vi "RRAM.vi"(5 "Other Fixed Voltage (V)":dbl=2.0, 7 "Pulse Width (us)":dbl=100.0, 8 "Mode":T1(tab), 9 "Stride":u16=1, 10 "Final address":u16, 11 "Initial address":u16) -> ()   [LabVIEW 2019]
uses:
  <vilib>/Utility/file.llb/Read Delimited Spreadsheet (I64).vi
  Globals.vi
  <vilib>/Utility/file.llb/Write Delimited Spreadsheet (DBL).vi
panel:
  in  "Addr hold time (s)":dbl=0.0005 caption="Time Target (s)" format="%#_6p"
  out "Current address":i32
  in  "FORM outfile":path=path "C:/Users/Murmann-Group/Documents/LabVIEW Data/NI-RRAM-Test-Setup/form.csv"
  out "FORM resistance (ohm)":dbl format="%#_6p"
  out "FORM WL voltage (V)":dbl
  out "FORM BL voltage (V)":dbl
  out "formed?":bool
  in  "SET target resistance (ohm)":dbl format="%#_6p"
  out "SET resistance (ohm)":dbl format="%#_6p"
  out "SET WL voltage (V)":dbl
  out "SET BL voltage (V)":dbl
  out "set?":bool
  in  "SET outfile":path=path "C:/Users/Murmann-Group/Documents/LabVIEW Data/NI-RRAM-Test-Setup/set.csv"
  in  "RESET target resistance (ohm)":dbl=50000.0 format="%#_6p"
  in  "RESET outfile":path=path "C:/Users/Murmann-Group/Documents/LabVIEW Data/NI-RRAM-Test-Setup/reset.csv"
  out "reset?":bool
  out "RESET SL voltage (V)":dbl
  out "RESET WL voltage (V)":dbl
  out "RESET resistance (ohm)":dbl format="%#_6p"
  in  "number of samples":i32=500
  in  "voltage level (V)":dbl=0.2 format="%#_6p"
  in  "settling time (s)":dbl=0.002 caption="Time Target (s)" format="%#_6p"
  in  "READ outfile":path=path "C:/Users/Murmann-Group/Documents/LabVIEW Data/NI-RRAM-Test-Setup/read.csv"
  out "read voltages (V)":dbl[](array[numeric]) format="%#_6p"
  out "currents (A)":dbl[](array[numeric]) format="%#_6p"
  out "resistances (ohm)":dbl[](array[numeric]) format="%#_6p"
  in  "Sweep Type":T2(ring)
  in  "Sweep outfile":path=path "C:/Users/Murmann-Group/Documents/LabVIEW Data/NI-RRAM-Test-Setup/sweep-vwl-set.csv"
  in  "Target infile":path=path "C:/Users/RSG/Desktop/NI-Skywater-Test-Setup/target.csv"
  in  "Target from file?":bool
  in  "Upper resistance (ohm)":dbl=50000.0 format="%#_6p"
  in  "Lower resistance (ohm)":dbl=40000.0 format="%#_6p"
  in  "Retention outfile":path=path "C:/Users/RSG/Desktop/NI-Skywater-Test-Setup/target.csv"
  in  "Perform retention test":bool
  out "target final resistance (ohm)":dbl format="%#_6p"
  out "target hit?":bool
  out "Current target (from file)":i64
  in  "Target outfile":path=path "C:/Users/RSG/Desktop/NI-Skywater-Test-Setup/target.csv"
  in  "CB type":u16(ring)=1 items=["1 bit/cell"=1, "2 bit/cell"=2, "3 bit/cell"=3, "4 bit/cell"=4]
  in  "Read Ranges (multi-bit)":dbl[](array[numeric])=[0.0, 7000.0, 28000.0, 85000.0, 1000000000.0] format="%#_6p"
  in  "Write Targets (multi-bit)":dbl[][](array[numeric])=[[0.0, 6000.0], [20000.0, 25000.0], [70000.0, 75000.0], [140000.0, 500000.0]] format="%#_6p"
  in  "Read Ranges (1b)":dbl[](array[numeric])=[0.0, 7000.0, 1000000000.0] format="%#_6p"
  in  "Write Targets (1b)":dbl[][](array[numeric])=[[9000.0, 11000.0], [100000.0, 10000000000.0]] format="%#_6p"
  in  "CB size":i32=32
  in  "CB offset":i32
  out "Checkerboard":T3(plugin-control)
  out "Confusion Matrix":i32[][](array[numeric])
  out "BER":dbl
  in  "endurance file":path
  in  "Cycles":i32
  # "Checkerboard Write"
  # "Checkerboard Read"
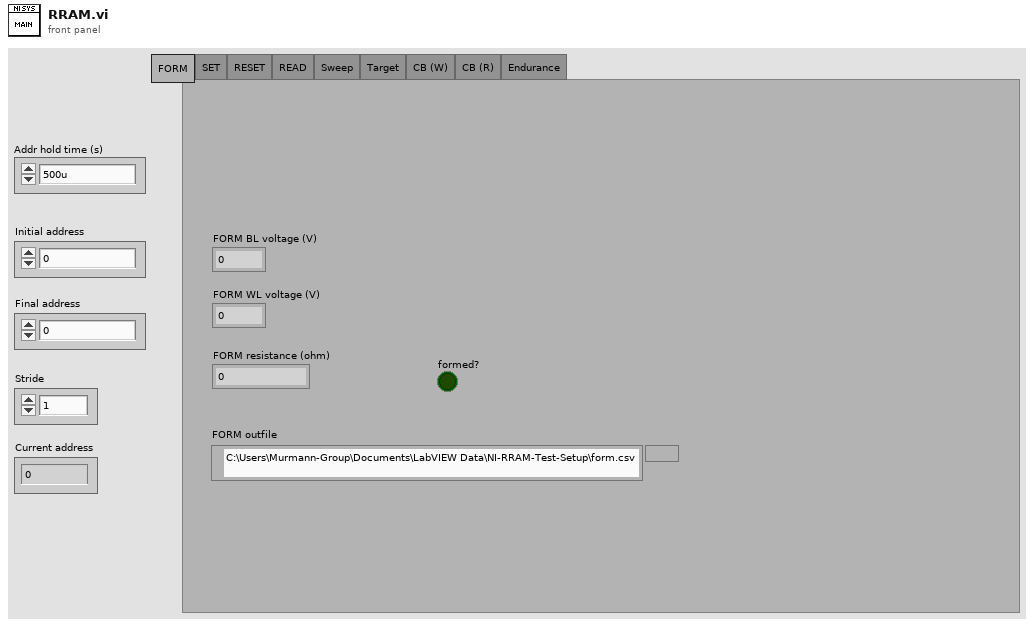
[diagram p1: front panel]
types:
  T1 = enum32{"FORM", "SET", "RESET", "READ", "Sweep", "Target", "CB (W)", "CB (R)", "Endurance"}
  T2 = enum16{"Sweep VWL SET", "Sweep VBL SET", "Sweep VWL RESET", "Sweep VSL RESET"}
  T3 = typedef "IMAQ Image.ctl" = refnum<image>
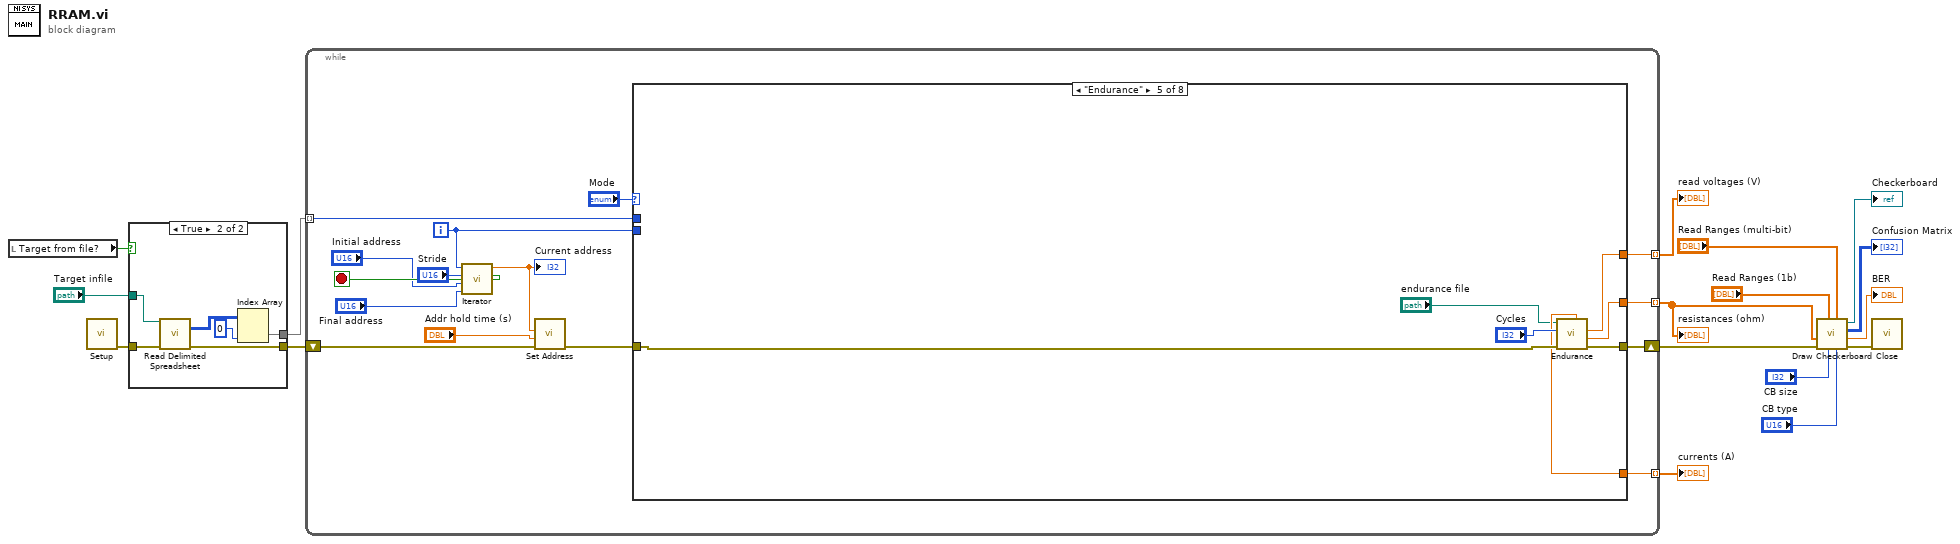
[diagram p0: block diagram]
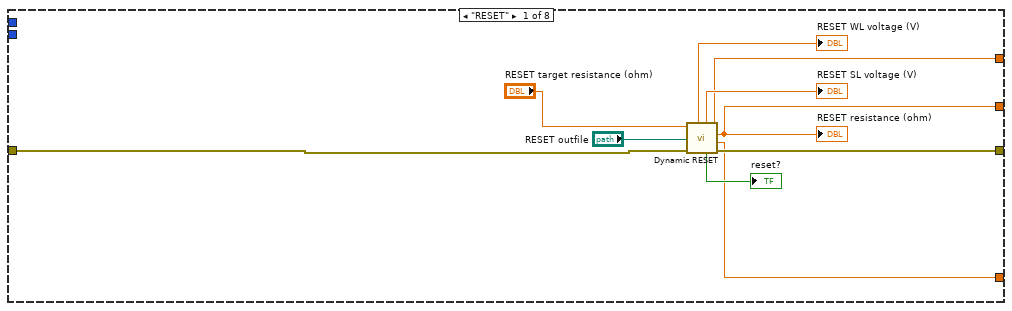
[diagram p3: hidden frame]
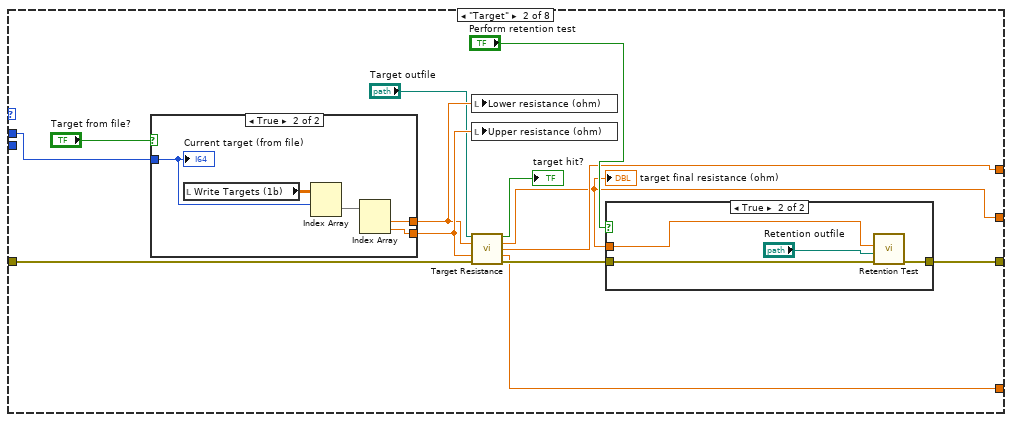
[diagram p4: hidden frame]
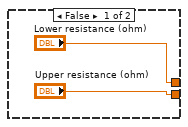
[diagram p5: hidden frame]
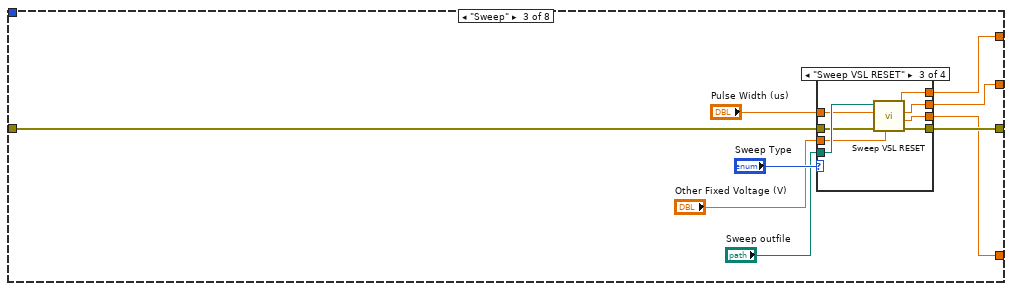
[diagram p7: hidden frame]
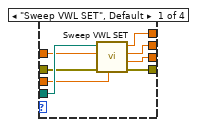
[diagram p8: hidden frame]
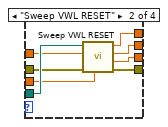
[diagram p9: hidden frame]
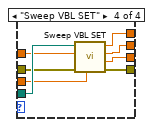
[diagram p10: hidden frame]
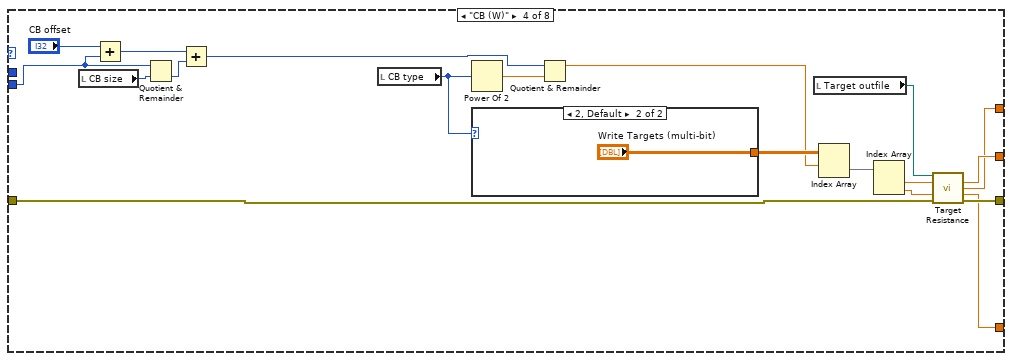
[diagram p11: hidden frame]
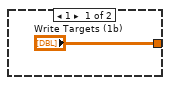
[diagram p12: hidden frame]
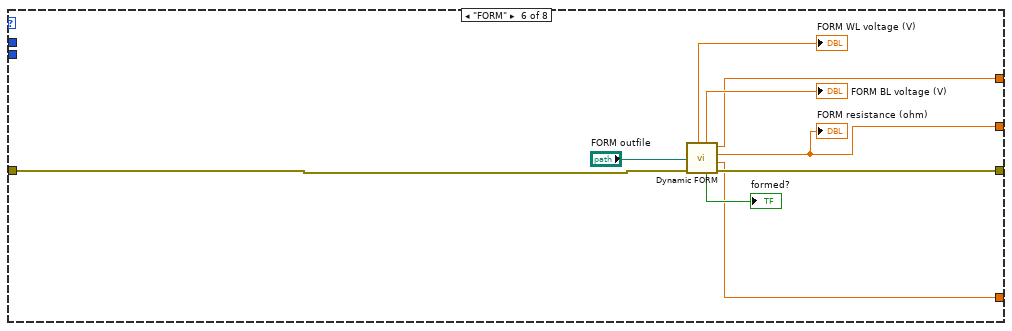
[diagram p13: hidden frame]
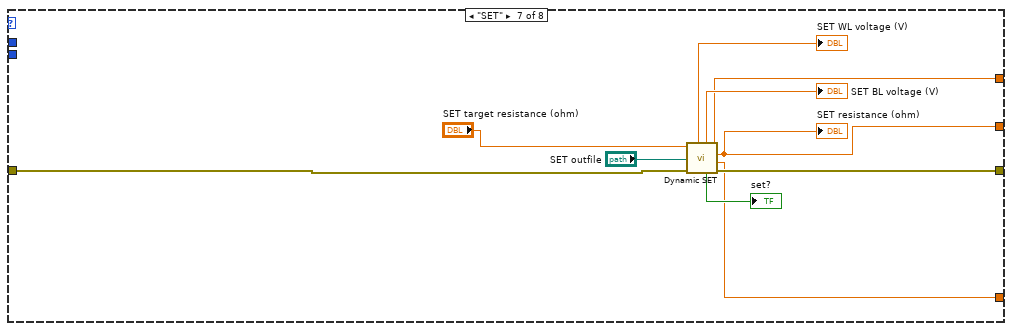
[diagram p14: hidden frame]
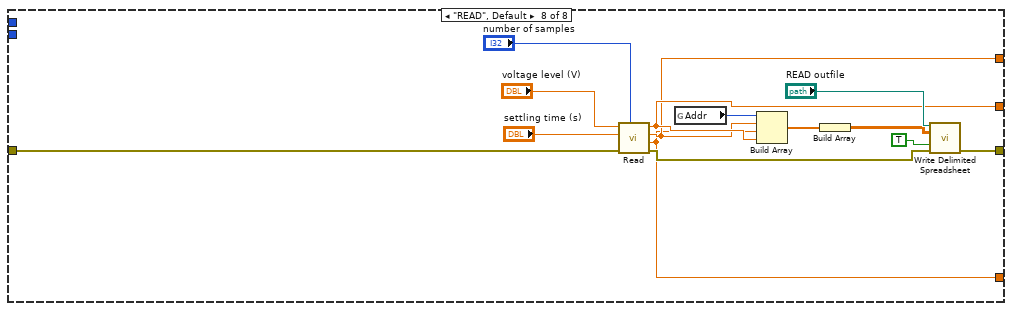
[diagram p15: hidden frame]
diagram:
  n1 = local read "Target from file?"() -> (w1:bool)
  n2 = call "Setup.vi"() -> ("error out"=w5:errorcluster)  [unwired: 10 in]
  n3 = case shown="True" w1 {
    tunnel: w5 -> [w18 w24]
    tunnel: [w18 w23] -> w4
    tunnel: "Target infile" -> [_ w22]
    tunnel: [_ w19] -> w2
    frame False {
    }
    frame True {
      n4 = call-poly <vilib>:"Read Delimited Spreadsheet.vi"("file path (dialog if empty)"=w22, "error in (no error)"=w24) -> ("all rows"=w21:i64[][], "error out"=w23:errorcluster)  [unwired: 8 in, 4 out]
      n5 = Index Array(array=w21, index (col)=0 ("disabled index (col)")) -> (element=w19:i64[])  [unwired: 1 in]
    }
  }
  n6 = while {
    shift-right: [w35] -> w16
    shift-left: w4 -> [w39]
    tunnel: [w28] -> w10 mode=indexing
    tunnel: [w27] -> w9 mode=indexing
    tunnel: [w26] -> w6 mode=indexing
    tunnel: w2 -> [w25] mode=indexing
    i -> [w30]
    stop <- w34 stop-if-true
    n7 = call "Iterator.vi"("Final Value"="Final address", "Initial Value"="Initial address", "Step"="Stride", "i"=w30) -> ("End Loop"=w34:bool, "Current Value"=w29:dbl)  [unwired: 6 in]
    "Current address" <- w29
    n8 = call "Set Address.vi"("error in (no error)"=w39, "hold time (s)"="Addr hold time (s)", "address"=w29) -> ("error out"=w36:errorcluster)  [unwired: 8 in]
    n9 = case shown="\"Endurance\"" "Mode" {
      tunnel: w36 -> [w48 w62 w81 w134 w142 w147 w162 w176]
      tunnel: [w49 w61 w82 w133 w141 w152 w161 w171] -> w35
      tunnel: w30 -> [_ _ _ w118 _ _ _ _]
      tunnel: [w42 w58 w79 w121 w140 w144 w156 w165] -> w28
      tunnel: [w40 w56 w78 w120 w138 w146 w154 w164] -> w27
      tunnel: [w41 w57 w80 w122 w139 w145 w155 w166] -> w26
      tunnel: w25 -> [_ w54 _ _ _ _ _ _]
      frame "RESET" {
        n10 = call "Dynamic RESET.vi"("error in (no error)"=w48, "RESET outfile"="RESET outfile", "target resistance"="RESET target resistance (ohm)") -> ("error out"=w49:errorcluster, "final current (A)"=w40:dbl, "final resistance (ohm)"=w41:dbl, "final read voltage (V)"=w42:dbl, "reset?"=→"reset?":bool, "SL voltage (V)"=→"RESET SL voltage (V)":dbl, "WL voltage (V)"=→"RESET WL voltage (V)":dbl)  [unwired: 2 in]
        "RESET resistance (ohm)" <- w41
      }
      frame "Target" {
        n11 = case shown="True" "Target from file?" {
          tunnel: ["Upper resistance (ohm)" w67] -> w52
          tunnel: ["Lower resistance (ohm)" w68] -> w51
          tunnel: w54 -> [_ w66]
          frame False {
          }
          frame True {
            n12 = local read "Write Targets (1b)"() -> (w65:dbl[][])
            n13 = Index Array(array=w65, index (row)=w66) -> (element=w69:dbl[])  [unwired: 1 in]
            n14 = Index Array(array=w69) -> (element #1=w68:dbl, element #2=w67:dbl)  [unwired: 2 in]
            "Current target (from file)" <- w66
          }
        }
        n15 = local write "Lower resistance (ohm)"(w51) -> ()
        n16 = local write "Upper resistance (ohm)"(w52) -> ()
        n17 = call "Target Resistance.vi"("Target outfile"="Target outfile", "Lower resistance (ohm)"=w51, "Upper resistance (ohm)"=w52, "error in (no error)"=w62) -> ("target hit?"=→"target hit?":bool, "final resistance (ohm)"=w57:dbl, "final voltage (V)"=w58:dbl, "final current (A)"=w56:dbl, "error out"=w60:errorcluster)  [unwired: 4 in, 3 out]
        "target final resistance (ohm)" <- w57
        n18 = case shown="True" "Perform retention test" {
          tunnel: w60 -> [w70 w74]
          tunnel: [w70 w73] -> w61
          tunnel: w57 -> [_ w71]
          frame False {
          }
          frame True {
            n19 = call "Retention Test.vi"("error in (no error)"=w74, "target outfile"="Retention outfile", "final resistance (ohm)"=w71) -> ("error out"=w73:errorcluster)  [unwired: 8 in]
          }
        }
      }
      frame "Sweep" {
        n20 = case shown="\"Sweep VSL RESET\"" "Sweep Type" {
          tunnel: [w84 w92 w103 w108] -> w82
          tunnel: w81 -> [w85 w93 w104 w109]
          tunnel: [w87 w95 w101 w112] -> w80
          tunnel: [w86 w94 w102 w111] -> w79
          tunnel: [w88 w96 w100 w110] -> w78
          tunnel: "Sweep outfile" -> [w91 w99 w107 w115]
          tunnel: "Pulse Width (us)" -> [w90 w98 w106 w114]
          tunnel: "Other Fixed Voltage (V)" -> [w89 w97 w105 w113]
          frame "Sweep VWL SET", Default {
            n21 = call "Sweep VWL SET.vi"("Other Fixed Voltage (V)"=w89, "error in (no error)"=w85, "Pulse Width (us)"=w90, "Sweep outfile"=w91) -> ("error out"=w84:errorcluster, "final current (A)"=w88:dbl, "final resistance (ohm)"=w87:dbl, "final voltage (V)"=w86:dbl)  [unwired: 4 in]
          }
          frame "Sweep VWL RESET" {
            n22 = call "Sweep VWL RESET.vi"("Other Fixed Voltage (V)"=w97, "error in (no error)"=w93, "Pulse Width (us)"=w98, "Sweep outfile"=w99) -> ("error out"=w92:errorcluster, "final current (A)"=w96:dbl, "final resistance (ohm)"=w95:dbl, "final voltage (V)"=w94:dbl)  [unwired: 4 in]
          }
          frame "Sweep VSL RESET" {
            n23 = call "Sweep VSL RESET.vi"("Other Fixed Voltage (V)"=w105, "error in (no error)"=w104, "Pulse Width (us)"=w106, "Sweep outfile"=w107) -> ("error out"=w103:errorcluster, "final current (A)"=w100:dbl, "final resistance (ohm)"=w101:dbl, "final voltage (V)"=w102:dbl)  [unwired: 4 in]
          }
          frame "Sweep VBL SET" {
            n24 = call "Sweep VBL SET.vi"("Other Fixed Voltage (V)"=w113, "error in (no error)"=w109, "Pulse Width (us)"=w114, "Sweep outfile"=w115) -> ("error out"=w108:errorcluster, "final current (A)"=w110:dbl, "final resistance (ohm)"=w112:dbl, "final voltage (V)"=w111:dbl)  [unwired: 4 in]
          }
        }
      }
      frame "CB (W)" {
        n25 = local read "CB size"() -> (w124:i32)
        n26 = Add(x="CB offset", y=w118) -> (x+y=w117:i32)
        n27 = Quotient & Remainder(x=w118, y=w124) -> (floor(x/y)=w123:i32)  [unwired: 1 out]
        n28 = Add(x=w117, y=w123) -> (x+y=w125:i32)
        n29 = local read "CB type"() -> (w130:u16)
        n30 = Power Of 2(x=w130) -> (2^x=w131:dbl)
        n31 = case shown="2, Default" w130 {
          tunnel: ["Write Targets (1b)" "Write Targets (multi-bit)"] -> w132
          frame 1 {
          }
          frame 2, Default {
          }
        }
        n32 = Quotient & Remainder(x=w125, y=w131) -> (x-y*floor(x/y)=w129:dbl)  [unwired: 1 out]
        n33 = local read "Target outfile"() -> (w116:path)
        n34 = Index Array(array=w132, index (row)=w129) -> (element=w128:dbl[])  [unwired: 1 in]
        n35 = Index Array(array=w128) -> (element #1=w127:dbl, element #2=w126:dbl)  [unwired: 2 in]
        n36 = call "Target Resistance.vi"("Target outfile"=w116, "Lower resistance (ohm)"=w127, "Upper resistance (ohm)"=w126, "error in (no error)"=w134) -> ("final resistance (ohm)"=w122:dbl, "final voltage (V)"=w121:dbl, "final current (A)"=w120:dbl, "error out"=w133:errorcluster)  [unwired: 4 in, 4 out]
      }
      frame "Endurance" {
        n37 = call "Endurance.vi"("error in (no error)"=w142, "Cycles"="Cycles", "endurance file"="endurance file") -> ("error out"=w141:errorcluster, "resistance (ohm)"=w139:dbl, "read voltage (V)"=w140:dbl, "current (A)"=w138:dbl)  [unwired: 4 in, 1 out]
      }
      frame "FORM" {
        n38 = call "Dynamic FORM.vi"("error in (no error)"=w147, "FORM outfile"="FORM outfile") -> ("error out"=w152:errorcluster, "final current (A)"=w146:dbl, "final resistance (ohm)"=w145:dbl, "final read voltage (V)"=w144:dbl, "formed?"=→"formed?":bool, "BL voltage (V)"=→"FORM BL voltage (V)":dbl, "WL voltage (V)"=→"FORM WL voltage (V)":dbl)  [unwired: 3 in]
        "FORM resistance (ohm)" <- w145
      }
      frame "SET" {
        n39 = call "Dynamic SET.vi"("error in (no error)"=w162, "SET outfile"="SET outfile", "target resistance"="SET target resistance (ohm)") -> ("error out"=w161:errorcluster, "final current (A)"=w154:dbl, "final resistance (ohm)"=w155:dbl, "final read voltage (V)"=w156:dbl, "set?"=→"set?":bool, "BL voltage (V)"=→"SET BL voltage (V)":dbl, "WL voltage (V)"=→"SET WL voltage (V)":dbl)  [unwired: 2 in]
        "SET resistance (ohm)" <- w155
      }
      frame "READ", Default {
        n40 = call "Read.vi"("number of samples"="number of samples", "error in (no error)"=w176, "settling time (s)"="settling time (s)", "voltage level (V)"="voltage level (V)") -> ("error out"=w172:errorcluster, "current (A)"=w164:dbl, "read voltage (V)"=w165:dbl, "resistance (ohm)"=w166:dbl)  [unwired: 4 in]
        n41 = global read "Globals.vi" "Addr"() -> (w163:u16)
        n42 = Build Array(w163, w165, w164, w166) -> (w168:dbl[])
        n43 = Build Array(w168) -> (w167:dbl[][])
        n44 = call-poly <vilib>:"Write Delimited Spreadsheet.vi"("file path (dialog if empty)"="READ outfile", "2D data"=w167, "append to file? (new file:F)"=TRUE, "error in (no error)"=w172) -> ("error out"=w171:errorcluster)  [unwired: 10 in, 1 out]
      }
    }
  }
  "read voltages (V)" <- w10
  "currents (A)" <- w9
  "resistances (ohm)" <- w6
  n45 = call "Draw Checkerboard.vi"("CB type"="CB type", "Resistance Read Ranges (multi-bit)"="Read Ranges (multi-bit)", "CB size"="CB size", "Resistance Read Ranges (1b)"="Read Ranges (1b)", "error in (no error)"=w16, "Resistances (ohm)"=w6) -> ("error out"=w8:errorcluster, "BER"=→"BER":dbl, "Confusion Matrix"=→"Confusion Matrix":i32[][], "Checkerboard"=→"Checkerboard":T3)  [unwired: 2 in]
  n46 = call "Close.vi"("error in (no error)"=w8) -> ()  [unwired: 11 in]
